vi "MyrioProject.vi"() -> ()   [LabVIEW 2017]
doc: "The myRIO Project template acquires acceleration data from the onboard accelerometer and displays the changes of acceleration values in a waveform chart."
uses:
  <vilib>/platform/TimedLoop/XDataNode/XDataNode.xnode
  <vilib>/Platform/TimedLoop/XDataNode/nitl_modes.ctl
  <vilib>/Platform/TimedLoop/XDataNode/XDNodeRunTimeDep.lvlib
  <vilib>/Platform/TimedLoop/XDataNode/wakeup.ctl
  <vilib>/Platform/TimedLoop/XDataNode/timing_clust.ctl
  <vilib>/myRIO/Common/Instrument Driver Framework/Utilities/typedefs/Generic FPGA Reference.ctl
  <vilib>/myRIO/Common/Instrument Driver Framework/Utilities/typedefs/myRIO v1.0 Reference.ctl
  <vilib>/myRIO/Common/Instrument Driver Framework/Utilities/typedefs/Hardware Version Enum.ctl
  <vilib>/myRIO/Common/Instrument Driver Framework/Utilities/typedefs/myRIO Generic Hardware Reference.ctl
  <vilib>/userdefined/High Color/nirio_resource_hc.ctl
  <vilib>/myRIO/Common/Instrument Driver Framework/myRIO v1.0/Encoder/typedefs/Encoder Channels Enum.ctl
  <vilib>/myRIO/Instrument Drivers/Onboard IO/Encoder/typedefs/Encoder Reference.ctl
  <vilib>/myRIO/Instrument Drivers/Onboard IO/Encoder/Encoder.lvlib
  <vilib>/myRIO/Common/Instrument Driver Framework/myRIO v1.0/Encoder/typedefs/Encoder Signal Mode.ctl
  <vilib>/myRIO/Instrument Drivers/Onboard IO/Encoder/vis/myRIO Encoder Open.xnode
  <vilib>/myRIO/Common/Instrument Driver Framework/myRIO v1.0/Encoder/vis/myRIO v1.1 Open Encoder.vi
  <vilib>/myRIO/Common/Instrument Driver Framework/myRIO v1.0/Encoder/vis/myRIO v1.0 Configure Encoder.vi
  <vilib>/myRIO/Common/Instrument Driver Framework/myRIO v1.0/Encoder/typedefs/Encoder Configuration v1.0.ctl
  <vilib>/myRIO/Instrument Drivers/Onboard IO/PWM/typedefs/PWM Configuration.ctl
  <vilib>/myRIO/Instrument Drivers/Onboard IO/PWM/PWM.lvlib
  <vilib>/myRIO/Common/Instrument Driver Framework/myRIO v1.0/PWM/typedefs/PWM Channels Enum.ctl
  <vilib>/myRIO/Instrument Drivers/Onboard IO/PWM/typedefs/PWM Reference.ctl
  <vilib>/myRIO/Instrument Drivers/Onboard IO/PWM/vis/myRIO PWM Open.xnode
  <vilib>/myRIO/Common/Instrument Driver Framework/myRIO v1.0/PWM/vis/myRIO v1.1 Open PWM.vi
  <vilib>/myRIO/Instrument Drivers/Onboard IO/AO/vis/Write.vi
  <vilib>/myRIO/Instrument Drivers/Onboard IO/AO/AO.lvlib
  <vilib>/myRIO/Express VI/Onboard Devices/Button/Button Express VI.xnode
  <vilib>/myRIO/Instrument Drivers/Onboard IO/DIO/DIO.lvlib
  <vilib>/myRIO/Common/Instrument Driver Framework/myRIO v1.0/DIO/typedefs/DIO Channels Enum.ctl
  <vilib>/myRIO/Common/Instrument Driver Framework/myRIO v1.0/DIO/typedefs/DIO Channels List.ctl
  <vilib>/myRIO/Instrument Drivers/Onboard IO/DIO/typedefs/DIO Reference.ctl
  <vilib>/myRIO/Instrument Drivers/Onboard IO/DIO/vis/myRIO DIO Open.xnode
  <vilib>/myRIO/Common/Instrument Driver Framework/Utilities/vis/Is FPGA Ref Available.vi
  <vilib>/myRIO/Common/Instrument Driver Framework/myRIO v1.0/DIO/vis/myRIO v1.1 Open DIO.vi
  <vilib>/myRIO/Express VI/Onboard IO/AO/AO Express VI.xnode
  <vilib>/myRIO/Common/Instrument Driver Framework/Utilities/typedefs/Analog Scaling Constants.ctl
  <vilib>/myRIO/Common/Instrument Driver Framework/Utilities/typedefs/Analog Scaling Constants List.ctl
  <vilib>/myRIO/Common/Instrument Driver Framework/myRIO v1.0/AO/typedefs/AO Channels Enum.ctl
  <vilib>/myRIO/Common/Instrument Driver Framework/myRIO v1.0/AO/typedefs/AO Channels List.ctl
  <vilib>/myRIO/Instrument Drivers/Onboard IO/AO/typedefs/AO Reference.ctl
  <vilib>/myRIO/Instrument Drivers/Onboard IO/AO/vis/myRIO AO Open.xnode
  <vilib>/myRIO/Common/Instrument Driver Framework/myRIO v1.0/AO/vis/myRIO v1.1 Open AO.vi
  <vilib>/myRIO/Express VI/Onboard IO/DO/DO Express VI.xnode
  <vilib>/myRIO/Instrument Drivers/Onboard IO/DIO/vis/Write.vi
  <vilib>/myRIO/Express VI/Onboard IO/PWM/PWM Express VI.xnode
  <vilib>/myRIO/Instrument Drivers/Onboard IO/PWM/vis/Set Duty Cycle and Frequency.vi
panel:
  in  "Duty Cycle 2":dbl(slide)=0.1 min=0.05 max=0.1 step=0.01 scale=0.02..0.1
  in  "Duty Cycle":dbl(slide)=0.1 min=0.05 max=0.1 step=0.01 scale=0.05..0.1
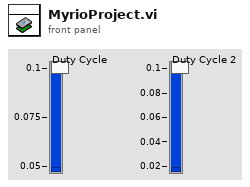
[diagram p1: front panel]
types:
  T1 = typedef "Encoder Signal Mode.ctl" = enum16{"Quadrature phase signal", "Step and direction signal"}
  T2 = typedef "PWM.lvlib/PWM Reference.ctl" = cluster{"myRIO Reference":T3, "PWM Channels Enum":T7, "PWM Configuration":T8}
  T3 = typedef "myRIO Generic Hardware Reference.ctl" = cluster{"myRIO Model":T4, "myRIO Hardware Reference":T5}
  T4 = typedef "Hardware Version Enum.ctl" = enum16{"Unknown", "myRIO-1900", "myRIO-1950", "roboRIO", "NI ELVIS RIO CM", "ELVIS III"}
  T5 = typedef "myRIO v1.0 Reference.ctl" = cluster{"Generic FPGA Reference":T6, "Allow multiple opens":bool}
  T6 = typedef "Generic FPGA Reference.ctl" = refnum<k20>
  T7 = typedef "PWM Channels Enum.ctl" = enum16{"Not Connected", "C/PWM0", "C/PWM1", "A/PWM0", "A/PWM1", "A/PWM2", "A/PWM3", "A/PWM4", "A/PWM5", "A/PWM6", "A/PWM7", "A/PWM8", "A/PWM9", "A/PWM10", "A/PWM11", "A/PWM12", "A/PWM13", "A/PWM14", "A/PWM15", "A/PWM16", "A/PWM17", "A/PWM18", "A/PWM19", "B/PWM0", "B/PWM1", "B/PWM2", "B/PWM3", "B/PWM4", "B/PWM5", "B/PWM6", "B/PWM7", "B/PWM8", "B/PWM9", "B/PWM10", "B/PWM11", "B/PWM12", "B/PWM13", "B/PWM14", "B/PWM15", "B/PWM16", "B/PWM17", "B/PWM18", "B/PWM19", "PWM/PWM0", "PWM/PWM1", "PWM/PWM2", "PWM/PWM3", "PWM/PWM4", "PWM/PWM5", "PWM/PWM6", "PWM/PWM7", "PWM/PWM8", "PWM/PWM9"}
  T8 = typedef "PWM.lvlib/PWM Configuration.ctl" = cluster{"Frequency":dbl, "Duty Cycle":dbl}
  T9 = typedef "Encoder.lvlib/Encoder Reference.ctl" = cluster{"myRIO Reference":T3, "Encoder Channels Enum":T10}
  T10 = typedef "Encoder Channels Enum.ctl" = enum16{"Not Connected", "C/ENC0", "C/ENC1", "A/ENC", "A/ENC0", "A/ENC1", "A/ENC2", "A/ENC3", "A/ENC4", "A/ENC5", "A/ENC6", "A/ENC7", "A/ENC8", "A/ENC9", "B/ENC", "B/ENC0", "B/ENC1", "B/ENC2", "B/ENC3", "B/ENC4", "B/ENC5", "B/ENC6", "B/ENC7", "B/ENC8", "B/ENC9", "DIO/ENC0", "DIO/ENC1", "DIO/ENC2", "DIO/ENC3", "DIO/ENC4"}
  T11 = typedef "XDNodeRunTimeDep.lvlib/timing_clust.ctl" = cluster{"Expected End [f-1]":u64, "Actual End [f-1]":u64, "Finished Late? [f-1]":bool, "Expected End [i-1]":u64, "Actual End [i-1]":u64, "Finished Late? [i-1]":bool, "Expected Start [i]":u64, "Actual Start [i]":u64, "Expected Start [f]":u64, "Actual Start [f]":u64, "Source Name":string, "Structure Name":string, "Period":i64, "Deadline":i64, "Offset":i64, "Start":i64, "Priority":i32, "Timeout":i32, "Mode":T12, "Wakeup Reason":T13, "Error":errorcluster, "Source Type":string, "Secondary Source Type":string, "Global End Time":u64, "Global Start Time":u64, "Frame Duration":u64, "Iteration Duration":u64, "Assigned CPU":i32, "I/O Scan Engine Mode":u32}
  T12 = typedef "XDNodeRunTimeDep.lvlib/nitl_modes.ctl" = enum32{"No Change", "Process missed periods, maintain original phase", "Discard missed periods, maintain original phase", "Process missed periods, ignore original phase", "Discard missed periods, ignore original phase"}
  T13 = typedef "XDNodeRunTimeDep.lvlib/wakeup.ctl" = enum32{"Normal", "Aborted", "Asynchronous wakeup", "Timing source error", "Timed loop error", "Timeout"}
  T14 = typedef "nirio_resource_hc.ctl" = tag
  T15 = typedef "DIO.lvlib/DIO Reference.ctl" = cluster{"myRIO Reference":T3, "DIO Channels List":T16}
  T16 = typedef "DIO Channels List.ctl" = T17[]
  T17 = typedef "DIO Channels Enum.ctl" = enum16{"Not Connected", "C/DIO0", "C/DIO1", "C/DIO2", "C/DIO3", "C/DIO4", "C/DIO5", "C/DIO6", "C/DIO7", "A/DIO0", "A/DIO1", "A/DIO2", "A/DIO3", "A/DIO4", "A/DIO5", "A/DIO6", "A/DIO7", "A/DIO8", "A/DIO9", "A/DIO10", "A/DIO11", "A/DIO12", "A/DIO13", "A/DIO14", "A/DIO15", "A/DIO16", "A/DIO17", "A/DIO18", "A/DIO19", "B/DIO0", "B/DIO1", "B/DIO2", "B/DIO3", "B/DIO4", "B/DIO5", "B/DIO6", "B/DIO7", "B/DIO8", "B/DIO9", "B/DIO10", "B/DIO11", "B/DIO12", "B/DIO13", "B/DIO14", "B/DIO15", "B/DIO16", "B/DIO17", "B/DIO18", "B/DIO19", "LED0", "LED1", "LED2", "LED3", "Button0", "DIO/DIO0", "DIO/DIO1", "DIO/DIO2", "DIO/DIO3", "DIO/DIO4", "DIO/DIO5", "DIO/DIO6", "DIO/DIO7", "DIO/DIO8", "DIO/DIO9", "SPI/CS0", "SPI/CS1", "SPI/CS2", "SPI/CS3", "LED RADIO (Green)", "LED RADIO (Red)", "LED COMM (Green)", "LED COMM (Red)", "LED MODE (Green)", "LED MODE (Red)"}
  T18 = typedef "AO.lvlib/AO Reference.ctl" = cluster{"myRIO Reference":T3, "AO Channel List":T19, "AO Scaling Constant List":T21}
  T19 = typedef "AO Channels List.ctl" = T20[]
  T20 = typedef "AO Channels Enum.ctl" = enum16{"Not Connected", "AudioOut/Left", "AudioOut/Right", "C/AO0", "C/AO1", "A/AO0", "A/AO1", "B/AO0", "B/AO1"}
  T21 = typedef "Analog Scaling Constants List.ctl" = T22[]
  T22 = typedef "Analog Scaling Constants.ctl" = cluster{"LSB Weight (Volts)":dbl, "Offset (Volts)":dbl, "Signed?":bool}
  T23 = cluster{"Double":dbl, dbl, "Numeric":dbl, "seconds since 1Jan1904":timestamp, "Double":dbl, dbl, "Numeric":dbl}
  T24 = cluster{"Double":dbl, "dbl Scaled Value":dbl, "Output":dbl, "seconds since 1Jan1904":timestamp, dbl, dbl, dbl}
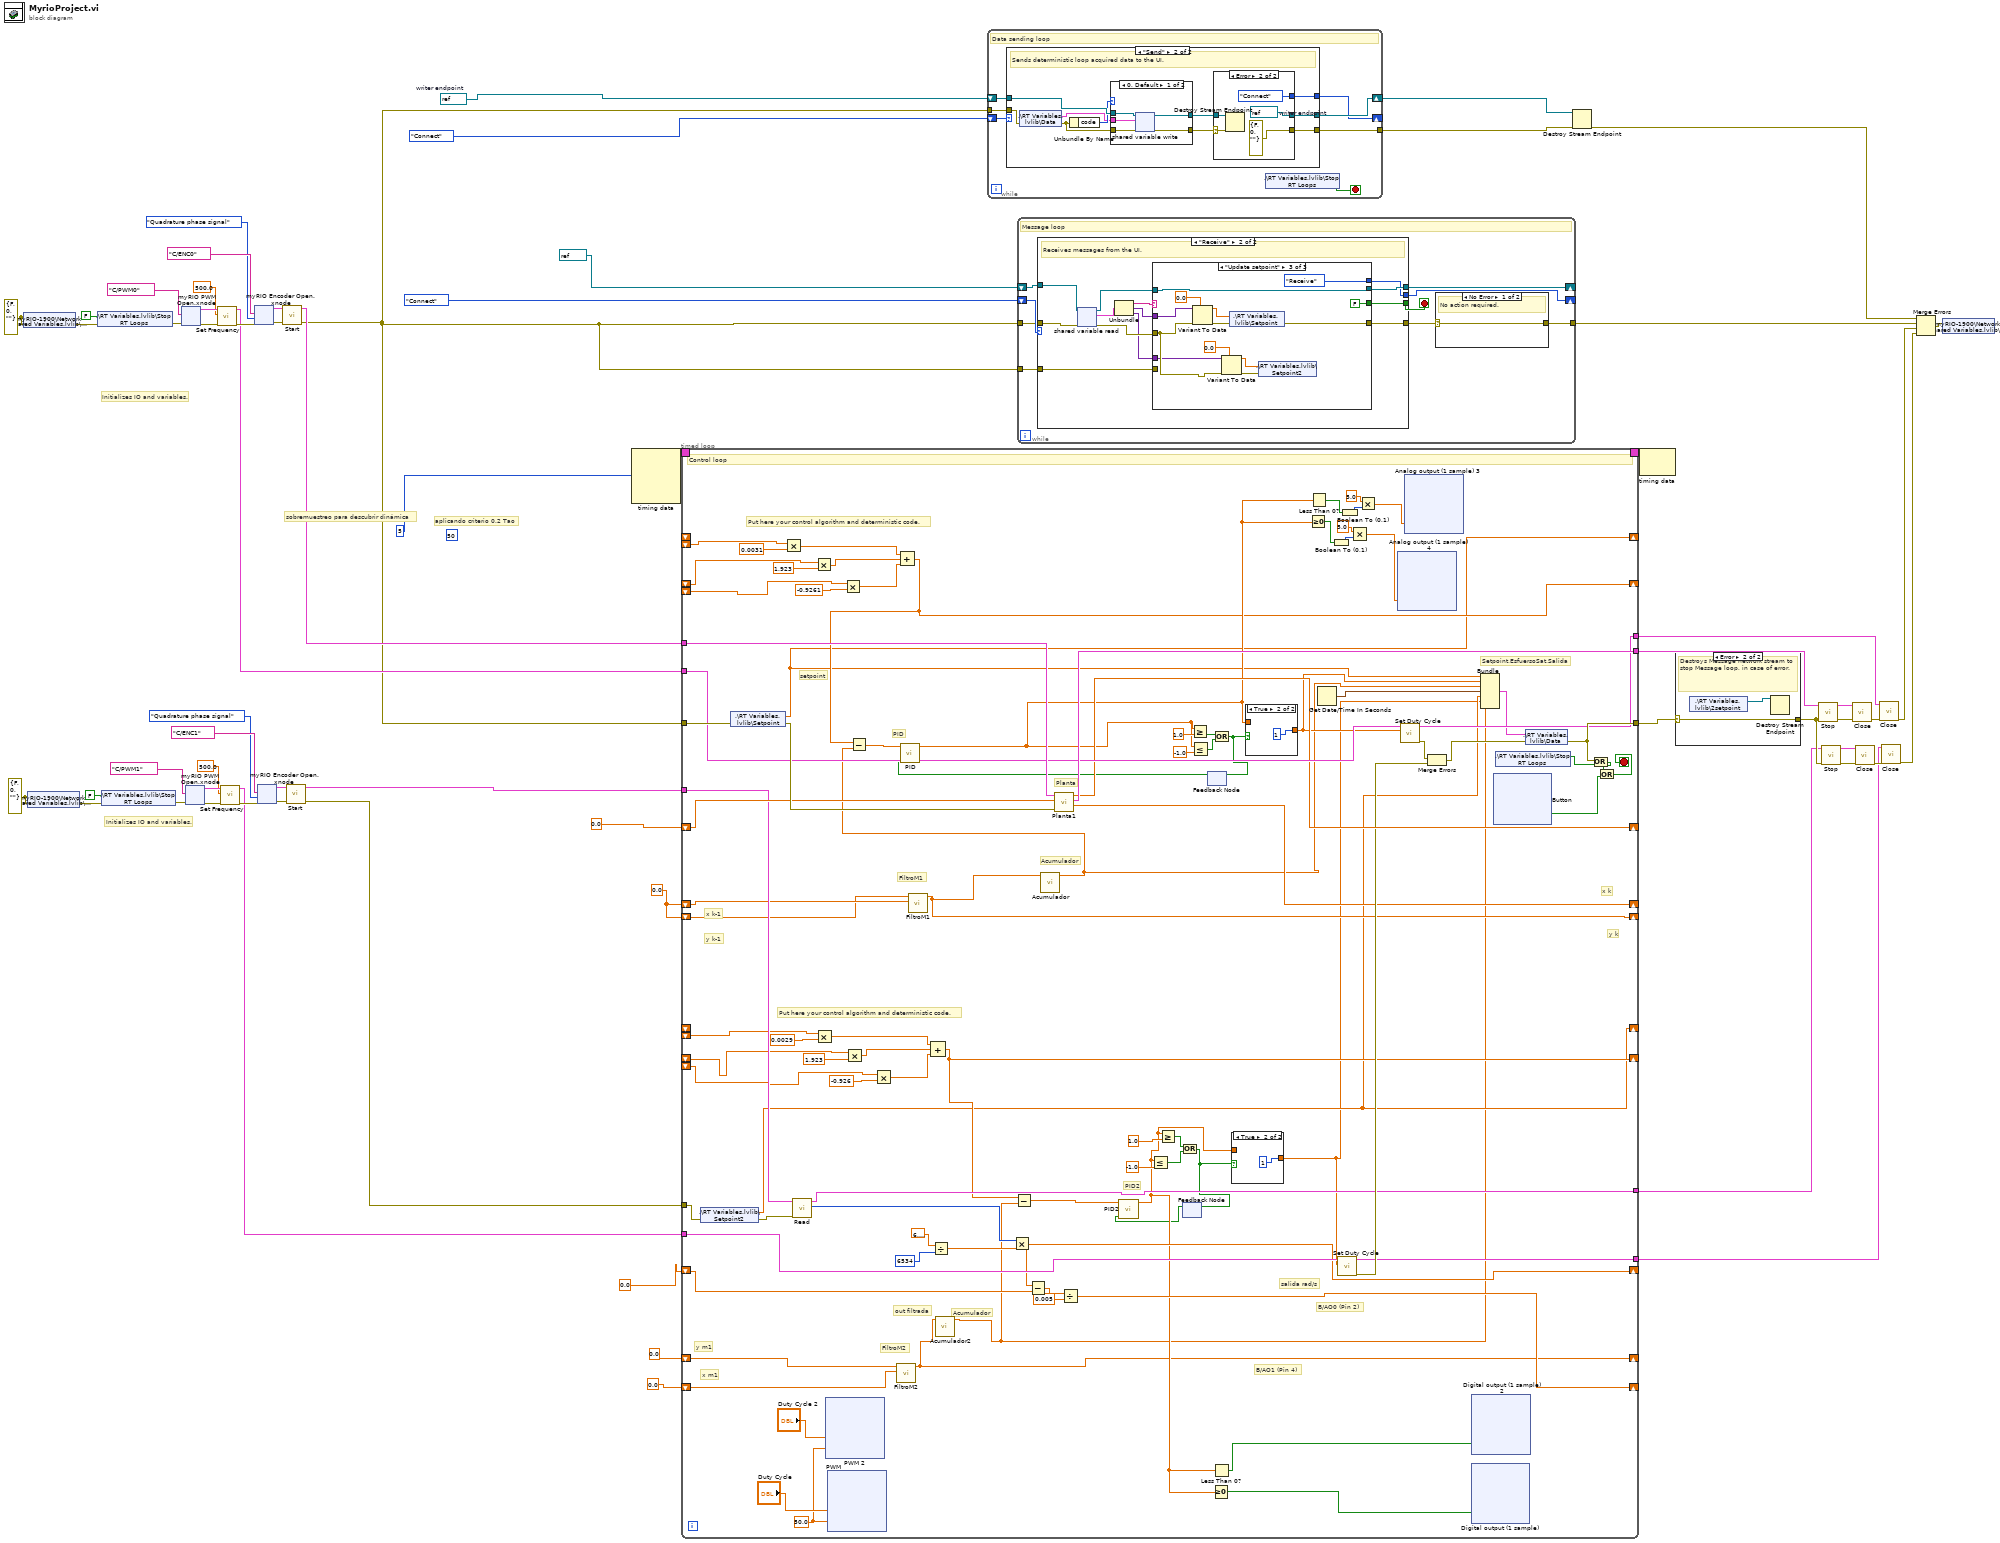
[diagram p0: block diagram]
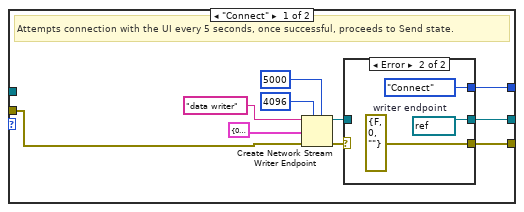
[diagram p3: hidden frame]
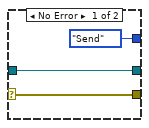
[diagram p4: hidden frame]
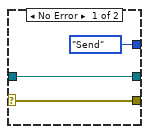
[diagram p5: hidden frame]
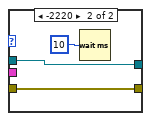
[diagram p6: hidden frame]
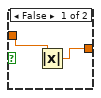
[diagram p7: hidden frame]
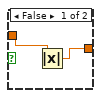
[diagram p8: hidden frame]
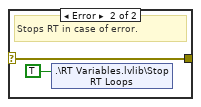
[diagram p9: hidden frame]
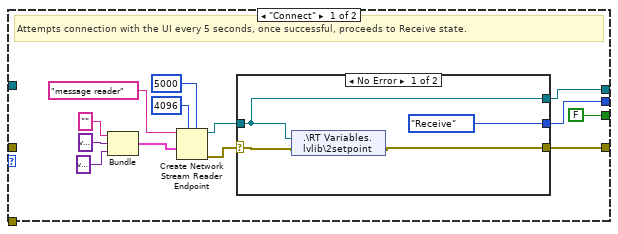
[diagram p10: hidden frame]
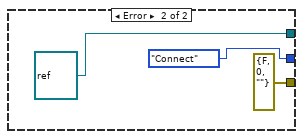
[diagram p11: hidden frame]
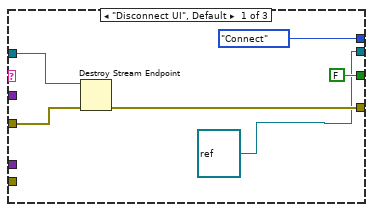
[diagram p12: hidden frame]
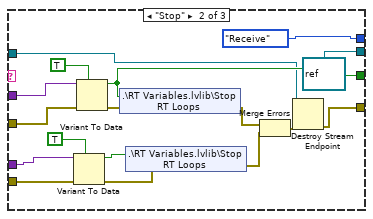
[diagram p13: hidden frame]
diagram:
  w2 = 0.0
  (unwired) 50
  w16 = refnum<k21> refnum  # writer endpoint
  w30 = errorcluster {"status"=FALSE, "code"=0, "source"=""} ("error IO")
  w52 = errorcluster {"status"=FALSE, "code"=0, "source"=""} ("error IO")
  # "aplicando criterio 0.2 Tao"
  # "sobremuestreo para descubrir dinámica"
  # "Initializes IO and variables."
  # "Initializes IO and variables."
  n1 = shared-variable "myRIO-1900\\Network Shared Variables.lvlib\\error IO"(w52, error in=w52) -> (error out=w53:errorcluster)
  n2 = shared-variable "myRIO-1900\\Network Shared Variables.lvlib\\error IO"(w30, error in=w30) -> (error out=w31:errorcluster)
  n3 = shared-variable ".\\RT Variables.lvlib\\Stop RT Loops"(FALSE ("Stop RT Loops"), error in=w53) -> (error out=w40:errorcluster)
  n4 = shared-variable ".\\RT Variables.lvlib\\Stop RT Loops"(FALSE ("Stop RT Loops"), error in=w31) -> (error out=w23:errorcluster)
  n5 = xnode "myRIO PWM Open.xnode"("error in (no error)"=w40, "Channel Name"=tag "C/PWM0") -> ("error out"=w42:errorcluster, "PWM Ref Out"=w41:T2)  [unwired: 1 in]
  n6 = xnode "myRIO PWM Open.xnode"("error in (no error)"=w23, "Channel Name"=tag "C/PWM1") -> ("error out"=w25:errorcluster, "PWM Ref Out"=w24:T2)  [unwired: 1 in]
  n7 = call <vilib>:"Set Frequency.vi"("error in (no error)"=w42, "Frequency [Hz]"=500.0, "PWM Ref In"=w41) -> ("error out"=w39:errorcluster, "PWM Ref Out"=w36:T2)  [unwired: 6 in]
  n8 = call <vilib>:"Set Frequency.vi"("error in (no error)"=w25, "Frequency [Hz]"=500.0, "PWM Ref In"=w24) -> ("error out"=w22:errorcluster, "PWM Ref Out"=w17:T2)  [unwired: 6 in]
  n9 = xnode "myRIO Encoder Open.xnode"("error in (no error)"=w39, "Channel Name"=tag "C/ENC0", "Encoder Signal Mode"=Encoder_Signal_Mode."Quadrature phase signal") -> ("error out"=w49:errorcluster, "Encoder Ref Out"=w48:T9)  [unwired: 2 in]
  n10 = xnode "myRIO Encoder Open.xnode"("error in (no error)"=w22, "Channel Name"=tag "C/ENC1", "Encoder Signal Mode"=Encoder_Signal_Mode."Quadrature phase signal") -> ("error out"=w28:errorcluster, "Encoder Ref Out"=w27:T9)  [unwired: 2 in]
  n11 = call <vilib>:"Start.vi"("error in (no error)"=w49, "Encoder Ref In"=w48) -> ("error out"=w8:errorcluster, "Encoder Ref Out"=w46:T9)  [unwired: 8 in]
  n12 = call <vilib>:"Start.vi"("error in (no error)"=w28, "Encoder Ref In"=w27) -> ("error out"=w19:errorcluster, "Encoder Ref Out"=w18:T9)  [unwired: 8 in]
  n13 = node-c288(i64 5 ("Period")) -> (w63:T11)  [unwired: 3 in]
  n14 = timed-loop {
    timing: w63 -> [_]
    timing-out: [_] -> w62
    tunnel: w8 -> [w157]
    tunnel: [w154] -> w51
    tunnel: w46 -> [w153]
    tunnel: [w152] -> w43
    tunnel: w36 -> [w151]
    tunnel: [w150] -> w35
    shift-right: [w147] -> _
    shift-left: 0.0 -> [w146]
    shift-right: [w118] -> _
    shift-left: 0.0 -> [w143]
    tunnel: w19 -> [w133]
    tunnel: w18 -> [w140]
    tunnel: w17 -> [w139]
    tunnel: [w135] -> w11
    tunnel: [w134] -> w10
    shift-right: [w65] -> _
    shift-left: 0.0 -> [w117]
    shift-right: [w119] -> _
    shift-left: 0.0 -> [w120]
    shift-right: [w100] -> _
    shift-left: w2 -> [w115]
    shift-right: [w114] -> _
    shift-left: w2 -> [w116]
    shift-right: [w87] -> _
    shift-left: _ -> [w90]
    shift-left: _ -> [w89]
    shift-right: [w70] -> _
    shift-left: _ -> [_]
    shift-left: _ -> [w88]
    shift-right: [w67] -> _
    shift-left: _ -> [_]
    shift-left: _ -> [w79]
    shift-right: [w76] -> _
    shift-left: _ -> [w78]
    shift-left: _ -> [w77]
    stop <- w124 stop-if-true
    w101 = 50.0 ("Frequency [Hz]")
    # "Setpoint,EsfuersoSat,Salida"
    # "setpoint"
    # "Acumulador"
    # "FiltroM2"
    # "PID2"
    # "Put here your control algorithm and deterministic code."
    # "Acumulador"
    # "Planta"
    # "y k"
    # "x k"
    # "FiltroM1"
    # "PID"
    # "x k-1"
    # "y k-1"
    # "out filtrada"
    # "x m1"
    # "y m1"
    # "salida rad/s"
    # "B/AO1 (Pin 4)"
    # "B/AO0 (Pin 2)"
    # "Put here your control algorithm and deterministic code."
    # "Control loop"
    n15 = shared-variable ".\\RT Variables.lvlib\\Setpoint2"(error in=w133) -> (w67:dbl, error out=w132:errorcluster)
    n16 = shared-variable ".\\RT Variables.lvlib\\Setpoint"(error in=w157) -> (w70:dbl, error out=w158:errorcluster)
    n17 = Multiply(x=w88, y=0.0031) -> (x*y=w92:dbl)
    n18 = call <vilib>:"Read.vi"("error in (no error)"=w132, "Encoder Ref In"=w140) -> ("Counter Value"=w142:i32, "Encoder Ref Out"=w135:T9)  [unwired: 5 in, 3 out]
    n19 = Multiply(x=w90, y=1.923) -> (x*y=w93:dbl)
    n20 = Multiply(x=w79, y=0.0029) -> (x*y=w81:dbl)
    n21 = xnode "PWM 2"("Duty Cycle"="Duty Cycle 2", "Frequency [Hz]"=w101) -> ()  [unwired: 1 in, 1 out]
    n22 = xnode "PWM"("Duty Cycle"="Duty Cycle", "Frequency [Hz]"=w101) -> ()  [unwired: 1 in, 1 out]
    n23 = Multiply(x=w89, y=-0.9261) -> (x*y=w91:dbl)
    n24 = Multiply(x=w78, y=1.923) -> (x*y=w82:dbl)
    n25 = Multiply(x=w77, y=-0.926) -> (x*y=w80:dbl)
    n26 = call "FiltroM2.vi"("Numeric 3"=w120, "Numeric in"=w117) -> ("Numeric out"=w65:dbl)  [unwired: 9 in]
    n27 = Compound Arithmetic op=ADD(w92, w93, w91) -> (w87:dbl)
    n28 = call "FiltroM1.vi"("Numeric 3"=w116, "Numeric in"=w115) -> ("Numeric out"=w100:dbl)  [unwired: 9 in]
    n29 = Compound Arithmetic op=ADD(w81, w82, w80) -> (w76:dbl)
    n30 = Divide(x=6.283185307179586, y=6534) -> (x/y=w141:dbl)
    n31 = call "Acumulador2.vi"("Numeric in"=w65) -> ("Numeric"=w64:dbl)  [unwired: 10 in]
    n32 = Multiply(x=w142, y=w141) -> (x*y=w118:dbl)
    n33 = Subtract(x=w76, y=w64) -> (x-y=w75:dbl)
    n34 = Subtract(x=w118, y=w143) -> (x-y=w144:dbl)
    n35 = call "Acumulador.vi"("Numeric in"=w100) -> ("Numeric"=w68:dbl)  [unwired: 10 in]
    n36 = Subtract(x=w87, y=w68) -> (x-y=w98:dbl)
    n37 = call "Planta1.vi"("error in (no error)"=w158, "Numeric in"=w146, "Encoder Ref Out in"=w153) -> ("velocidad"=w114:dbl, "Encoder Ref Out out"=w152:T9, "angulo"=w147:dbl)  [unwired: 6 in]
    n38 = Divide(x=w144, y=0.005) -> (x/y=w119:dbl)
    n39 = feedback #1() -> (w72:bool)  [unwired: 1 in]
    n40 = call "PID2.vi"("Boolean"=w72, "Numeric in"=w75) -> ("Numeric out"=w74:dbl)  [unwired: 9 in]
    n41 = Less Or Equal?(x=w74, y=-1.0) -> (x <= y?=w106:bool)
    n42 = Greater Or Equal?(x=w74, y=1.0) -> (x >= y?=w107:bool)
    n43 = Or(x=w107, y=w106) -> (x .or. y?=w71:bool)
    n44 = feedback-in #1(w71) -> ()
    n45 = feedback #2() -> (w86:bool)  [unwired: 1 in]
    n46 = call "PID.vi"("Boolean"=w86, "Numeric in"=w98) -> ("Numeric out"=w97:dbl)  [unwired: 9 in]
    n47 = Greater Or Equal?(x=w97, y=1.0) -> (x >= y?=w113:bool)
    n48 = Less Or Equal?(x=w97, y=-1.0) -> (x <= y?=w111:bool)
    n49 = Greater Or Equal To 0?(x=w74) -> (x >= 0?=w105:bool)
    n50 = Less Than 0?(x=w74) -> (x < 0?=w104:bool)
    n51 = Or(x=w113, y=w111) -> (x .or. y?=w73:bool)
    n52 = feedback-in #2(w73) -> ()
    n53 = case shown="True" w71 {
      tunnel: [w299 1] -> w66
      tunnel: w74 -> [w300 _]
      frame False {
        n54 = Absolute Value(x=w300) -> (abs(x)=w299:dbl)
      }
      frame True {
      }
    }
    n55 = case shown="True" w73 {
      tunnel: [w302 1] -> w69
      tunnel: w97 -> [w303 _]
      frame False {
        n56 = Absolute Value(x=w303) -> (abs(x)=w302:dbl)
      }
      frame True {
      }
    }
    n57 = Greater Or Equal To 0?(x=w97) -> (x >= 0?=w126:bool)
    n58 = Less Than 0?(x=w97) -> (x < 0?=w129:bool)
    n59 = Get Date/Time In Seconds() -> (seconds since 1Jan1904=w156:timestamp)
    n60 = Boolean To (0,1)(Boolean=w126) -> (0, 1=w127:i16)
    n61 = call <vilib>:"Set Duty Cycle.vi"("Duty Cycle"=w66, "PWM Ref In"=w139) -> ("error out"=w138:errorcluster, "PWM Ref Out"=w134:T2)  [unwired: 7 in]
    n62 = Boolean To (0,1)(Boolean=w129) -> (0, 1=w130:i16)
    n63 = Multiply(x=5.0, y=w127) -> (x*y=w121:dbl)
    n64 = Multiply(x=5.0, y=w130) -> (x*y=w122:dbl)
    n65 = xnode "Analog output (1 sample) 4"("C/AO1 (AO1)"=w121) -> ()  [unwired: 1 in, 1 out]
    n66 = call <vilib>:"Set Duty Cycle.vi"("Duty Cycle"=w69, "PWM Ref In"=w151) -> ("error out"=w137:errorcluster, "PWM Ref Out"=w150:T2)  [unwired: 7 in]
    n67 = xnode "Analog output (1 sample) 3"("C/AO0 (AO0)"=w122) -> ()  [unwired: 1 in, 1 out]
    n68 = Merge Errors(w137, w138) -> (w136:errorcluster)
    n69 = xnode "Digital output (1 sample)"("A/DIO0 (Pin 11)"=w105) -> ()  [unwired: 1 in, 1 out]
    n70 = xnode "Digital output (1 sample) 2"("A/DIO1 (Pin 13)"=w104) -> ()  [unwired: 1 in, 1 out]
    n71 = Bundle("Double"=w70, w69, "Numeric"=w68, "seconds since 1Jan1904"=w156, "Double"=w67, w66, "Numeric"=w64) -> (w149:T23)  [unwired: 1 in]
    n72 = xnode "Button"() -> ("Value"=w123:bool)  [unwired: 1 in, 1 out]
    n73 = shared-variable ".\\RT Variables.lvlib\\Stop RT Loops"() -> (w155:bool)  [unwired: 1 in, 1 out]
    n74 = shared-variable ".\\RT Variables.lvlib\\Data"(w149, error in=w136) -> (error out=w154:errorcluster)
    n75 = Or(x=w154, y=w155) -> (x .or. y?=w125:bool)
    n76 = Or(x=w125, y=w123) -> (x .or. y?=w124:bool)
  }
  n77 = while {
    shift-right: [w420] -> w58
    shift-left: w16 -> [w418]
    tunnel: [w419] -> w59
    tunnel: w8 -> [w417]
    shift-right: [w416] -> _
    shift-left: enum16{"Connect", "Send"}."Connect" ("Message states") -> [w421]
    stop <- w422 stop-if-true
    # "Data sending loop"
    n78 = case shown="\"Send\"" w421 {
      tunnel: [w426 w441] -> w419
      tunnel: [w424 w439] -> w420
      tunnel: [w430 w442] -> w416
      tunnel: w418 -> [_ w448]
      tunnel: w417 -> [w427 w447]
      frame "Connect" {
        # "Attempts connection with the UI every 5 seconds, once successful, proceeds to Send state."
        n79 = Create Network Stream Writer Endpoint(5:5000 ("timeout in ms (-1)"), 7:4096 ("writer buffer size"), 8:w427, 9:T24 {"Double"=0.0, "dbl Scaled Value"=0.0, "Output"=0.0, "seconds since 1Jan1904"=timestamp(0 s since 1904-01-01), 0.0, 0.0, 0.0} ("Data"), 11:"data writer" ("writer name")) -> (0:w428:errorcluster, 3:w425:refnum<k21>)  [unwired: 2 in]
        n80 = case shown="Error" w428 {
          selector: w428 -> [w433 _]
          tunnel: [enum16{"Connect", "Send"}."Send" ("Message states") enum16{"Connect", "Send"}."Connect" ("Message states")] -> w430
          tunnel: [w433 errorcluster {"status"=FALSE, "code"=0, "source"=""} ("error IO")] -> w426
          tunnel: w425 -> [w435 _]
          tunnel: [w435 w436] -> w424
          frame No Error {
          }
          frame Error {
            w436 = refnum<k21> refnum  # writer endpoint
          }
        }
      }
      frame "Send" {
        # "Sends deterministic loop acquired data to the UI."
        n81 = shared-variable ".\\RT Variables.lvlib\\Data"(error in=w447) -> (w444:T24, error out=w446:errorcluster)
        n82 = Unbundle By Name(w446) -> ("code"=w445:i32)
        n83 = case shown="0, Default" w445 {
          tunnel: [w461 w463] -> w443
          tunnel: [w460 w462] -> w440
          tunnel: w448 -> [w459 w462]
          tunnel: w446 -> [w458 w463]
          tunnel: w444 -> [w457 _]
          frame 0, Default {
            n84 = shared-variable-write(w459, w458, w457) -> (w460:refnum<k21>, w461:errorcluster)  [unwired: 1 in, 1 out]
          }
          frame -2220 {
            n85 = Wait (ms)(milliseconds to wait=u32 10) -> ()  [unwired: 1 out]
          }
        }
        n86 = case shown="Error" w443 {
          selector: w443 -> [w451 w455]
          tunnel: [enum16{"Connect", "Send"}."Send" ("Message states") enum16{"Connect", "Send"}."Connect" ("Message states")] -> w442
          tunnel: [w451 errorcluster {"status"=FALSE, "code"=0, "source"=""} ("error IO")] -> w441
          tunnel: w440 -> [w449 w454]
          tunnel: [w449 w452] -> w439
          frame No Error {
          }
          frame Error {
            w452 = refnum<k21> refnum  # writer endpoint
            n87 = Destroy Stream Endpoint(8:w455, 11:w454) -> ()  [unwired: 1 out]
          }
        }
      }
    }
    n88 = shared-variable ".\\RT Variables.lvlib\\Stop RT Loops"() -> (w422:bool)  [unwired: 1 in, 1 out]
  }
  n89 = while {
    tunnel: [w467] -> w55
    shift-right: [w472] -> _
    shift-left: refnum<k21> refnum ("reader endpoint") -> [w470]
    shift-right: [w471] -> _
    shift-left: enum16{"Connect", "Receive"}."Connect" ("Message states") -> [w473]
    tunnel: w8 -> [w469]
    tunnel: w8 -> [w465]
    stop <- w466 stop-if-true
    # "Message loop"
    n90 = case shown="\"Receive\"" w473 {
      tunnel: [w480 w505] -> w468
      tunnel: [w478 w506] -> w472
      tunnel: [w487 w502] -> w471
      tunnel: w470 -> [_ w500]
      tunnel: w469 -> [_ w504]
      tunnel: [FALSE ("Stop RT Loops") w503] -> w466
      tunnel: w465 -> [_ w497]
      frame "Connect" {
        # "Attempts connection with the UI every 5 seconds, once successful, proceeds to Receive state."
        n91 = Bundle("", variant, variant) -> (w483:cluster{string, variant, variant})  [unwired: 1 in]
        n92 = Create Network Stream Reader Endpoint(5:5000 ("timeout in ms (-1)"), 7:4096 ("reader buffer size"), 9:w483, 11:"message reader" ("reader name")) -> (0:w482:errorcluster, 3:w477:refnum<k21>)  [unwired: 3 in]
        n93 = case shown="No Error" w482 {
          selector: w482 -> [w491 _]
          tunnel: [enum16{"Connect", "Receive"}."Receive" ("Message states") enum16{"Connect", "Receive"}."Connect" ("Message states")] -> w487
          tunnel: [w490 errorcluster {"status"=FALSE, "code"=0, "source"=""} ("error IO")] -> w480
          tunnel: [w492 refnum<k21> refnum ("reader endpoint")] -> w478
          tunnel: w477 -> [w492 _]
          frame No Error {
            n94 = shared-variable ".\\RT Variables.lvlib\\2setpoint"(w492, error in=w491) -> (error out=w490:errorcluster)
          }
          frame Error {
          }
        }
      }
      frame "Receive" {
        # "Receives messages from the UI."
        n95 = shared-variable-read(w500, w504) -> (w499:refnum<k21>, w507:errorcluster, w501:cluster{string, variant, variant})  [unwired: 1 in, 1 out]
        n96 = Unbundle(w501) -> (w509:string, w508:variant, w498:variant)
        n97 = case shown="\"Update setpoint\"" w509 {
          tunnel: w508 -> [_ w530 w545]
          tunnel: w507 -> [w513 w532 w534]
          tunnel: [w512 w527 w541] -> w505
          tunnel: [refnum<k21> refnum ("reader endpoint") refnum<k21> refnum ("reader endpoint") w540] -> w506
          tunnel: w499 -> [w511 w526 w540]
          tunnel: [FALSE ("Stop RT Loops") w529 FALSE ("Stop RT Loops")] -> w503
          tunnel: [enum16{"Connect", "Receive"}."Connect" ("Message states") enum16{"Connect", "Receive"}."Receive" ("Message states") enum16{"Connect", "Receive"}."Receive" ("Message states")] -> w502
          tunnel: w498 -> [_ w522 w533]
          tunnel: w497 -> [_ w521 _]
          frame "Disconnect UI", Default {
            n98 = Destroy Stream Endpoint(8:w513, 11:w511) -> (0:w512:errorcluster)
          }
          frame "Stop" {
            n99 = Variant To Data(error in=w521, type=TRUE ("Stop RT Loops"), Variant=w522) -> (data=w519:bool, error out=w523:errorcluster)
            n100 = Variant To Data(error in=w532, type=TRUE ("Stop RT Loops"), Variant=w530) -> (data=w529:bool, error out=w531:errorcluster)
            n101 = shared-variable ".\\RT Variables.lvlib\\Stop RT Loops"(w529, error in=w531) -> (error out=w517:errorcluster)
            n102 = shared-variable ".\\RT Variables.lvlib\\Stop RT Loops"(w519, error in=w523) -> (error out=w518:errorcluster)
            n103 = Merge Errors(w517, w518) -> (w516:errorcluster)
            n104 = Destroy Stream Endpoint(8:w516, 11:w526) -> (0:w527:errorcluster)
          }
          frame "Update setpoint" {
            n105 = Variant To Data(error in=w534, type=0.0, Variant=w545) -> (data=w543:dbl, error out=w542:errorcluster)
            n106 = Variant To Data(error in=w534, type=0.0, Variant=w533) -> (data=w536:dbl, error out=w535:errorcluster)
            n107 = shared-variable ".\\RT Variables.lvlib\\Setpoint"(w543, error in=w542) -> (error out=w541:errorcluster)
            n108 = shared-variable ".\\RT Variables.lvlib\\Setpoint2"(w536, error in=w535) -> ()  [unwired: 1 out]
          }
        }
      }
    }
    n109 = case shown="No Error" w468 {
      selector: w468 -> [w474 w475]
      tunnel: [w474 w475] -> w467
      frame No Error {
        # "No action required."
      }
      frame Error {
        # "Stops RT in case of error."
        n110 = shared-variable ".\\RT Variables.lvlib\\Stop RT Loops"(TRUE ("Stop RT Loops")) -> ()  [unwired: 1 in, 1 out]
      }
    }
  }
  n111 = Destroy Stream Endpoint(8:w59, 11:w58) -> (0:w56:errorcluster)
  n112 = node-c288(w62) -> ()  [unwired: 1 out]
  n113 = case shown="Error" w51 {
    selector: w51 -> [w546 w547]
    tunnel: [w546 w547] -> w12
    frame No Error {
      # "No action required."
    }
    frame Error {
      # "Destroys Message network stream to stop Message loop, in case of error."
      n114 = shared-variable ".\\RT Variables.lvlib\\2setpoint"() -> (w548:refnum<k21>)  [unwired: 1 in, 1 out]
      n115 = Destroy Stream Endpoint(11:w548) -> ()  [unwired: 1 in, 1 out]
    }
  }
  n116 = call <vilib>:"Stop.vi"("error in (no error)"=w12, "Encoder Ref In"=w43) -> ("error out"=w44:errorcluster, "Encoder Ref Out"=w45:T9)  [unwired: 8 in]
  n117 = call <vilib>:"Stop.vi"("error in (no error)"=w12, "Encoder Ref In"=w11) -> ("error out"=w14:errorcluster, "Encoder Ref Out"=w15:T9)  [unwired: 8 in]
  n118 = call <vilib>:"Close.vi"("error in (no error)"=w44, "Encoder Ref In"=w45) -> ("error out"=w38:errorcluster)  [unwired: 9 in]
  n119 = call <vilib>:"Close.vi"("error in (no error)"=w14, "Encoder Ref In"=w15) -> ("error out"=w13:errorcluster)  [unwired: 9 in]
  n120 = call <vilib>:"Close.vi"("error in (no error)"=w38, "PWM Ref In"=w35) -> ("error out"=w37:errorcluster)  [unwired: 9 in]
  n121 = call <vilib>:"Close.vi"("error in (no error)"=w13, "PWM Ref In"=w10) -> ("error out"=w9:errorcluster)  [unwired: 9 in]
  n122 = Merge Errors(w56, w55, w37, w9) -> (w54:errorcluster)
  n123 = shared-variable "myRIO-1900\\Network Shared Variables.lvlib\\error IO"(w54) -> ()  [unwired: 1 in, 1 out]
